vi "Set Indicator.vi"(8 "error in (no error)":errorcluster, 10 "Indicater":i32, 11 "Panel_UI in":refnum<class "Panel_UI.lvclass">) -> (0 "error out":errorcluster, 3 "Panel_UI out":refnum<class "Panel_UI.lvclass">)   [LabVIEW 2015, in "Panel_UI.lvclass"]
uses:
  Panel_UI.lvclass
  Panel_UI.lvclass/Panel_UI.ctl
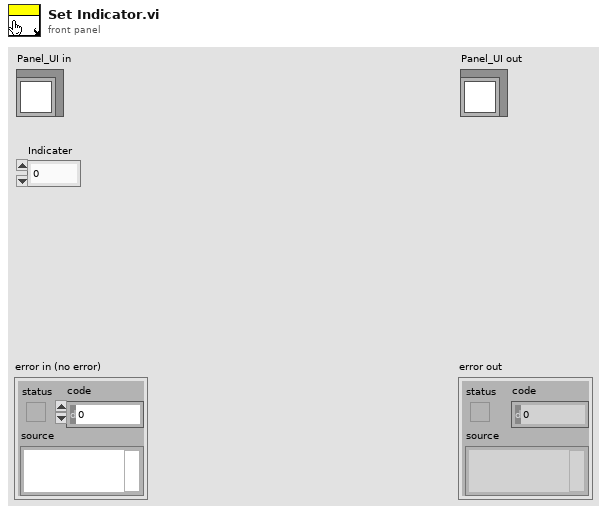
[diagram p1: front panel]
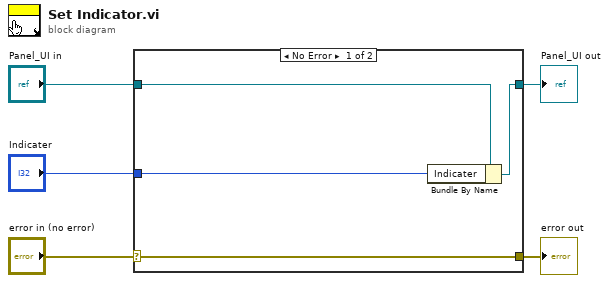
[diagram p0: block diagram]
diagram:
  n1 = case shown="No Error" "error in (no error)" {
    selector: "error in (no error)" -> [w9 w10]
    tunnel: [w9 w10] -> w4
    tunnel: [w7 w11] -> w2
    tunnel: "Panel_UI in" -> [w8 w11]
    tunnel: "Indicater" -> [w6 _]
    frame No Error {
      n2 = Bundle By Name(cluster=w8, "Indicater"=w6) -> (w7:refnum<class "Panel_UI.lvclass">)
    }
    frame Error {
    }
  }
  "error out" <- w4
  "Panel_UI out" <- w2
